vi "Outputs SW Set.vi"(7 "Current Time":timestamp format="%<%x %.3X>T", 8 "Grabber Config":T1={"Grabber Ver"=0, "CAN"={"ID"=0, "Bus"=""}, "Output"={"Type"=enum."Counter-Clockwise", "Neutral"=enum."Override to Coast", "Max"={"FWD"=1.0, "REV"=-1.0}, "Min"={"FWD"=0.0, "REV"=0.0}, "OL Ramp Rate (S)"=0.0, "Dead Band"=0.0}, "StatorLimit"={"Enable"=FALSE, "Current Limit"=0.0, "Threshold Current"=0.0, "Threshold Time"=0.0}} {"Output"."Min"."REV" format="%.2f"; "Output"."Min"."FWD" format="%.2f"; "Output"."Max"."REV" format="%.2f"; "Output"."Max"."FWD" format="%.2f"}, 9 "SW Config":T8={"GrabberSW Ver"=0, "Intake Speed"=0.2, "Eject Speed"=0.2, "Current Limit Velocity"=0, "Current Limit"=6.0, "Current Starting"=20.0, "Max Full Time(S)"=20.0}, 10 "Sensor Values":T10, 11 "SW Output":T9) -> (3 "SW Output Out":T9)   [LabVIEW 2020, in "Grabber_ACT.lvlib"]
uses:
  Grabber_ACT.lvlib
  Shared Code/TypeDefs/Cluster_Grabber HW Outputs.ctl
  Shared Code/TypeDefs/Cluster_FX Sensor Values.ctl
  Shared Code/TypeDefs/Cluster_FX CloseLoop Values.ctl
  Shared Code/TypeDefs/Cluster_FX Current Values.ctl
  Shared Code/TypeDefs/Cluster_Grabber_SW Outputs.ctl
  Shared Code/TypeDefs/Cluster_Grabber_Config SW Values.ctl
  Shared Code/TypeDefs/Cluster_Grabber_Config FX Values.ctl
  Shared Code/TypeDefs/Cluser_CAN Data.ctl
  Shared Code/TypeDefs/Cluster_Config Motor Output.ctl
  <vilib>/Rock Robotics/WPI/ThirdParty/Phoenix-LabVIEW/Motor Controller/Controls/CTRE_Phoenix_MotorControl_TalonFXInvertType.ctl
  <vilib>/Rock Robotics/WPI/ThirdParty/Phoenix-LabVIEW/Motor Controller/Controls/CTRE_Phoenix_MotorControl_NeutralMode.ctl
  Shared Code/TypeDefs/Cluster_FWD  REV Values.ctl
  Shared Code/TypeDefs/Cluser_Config_Current Limits.ctl
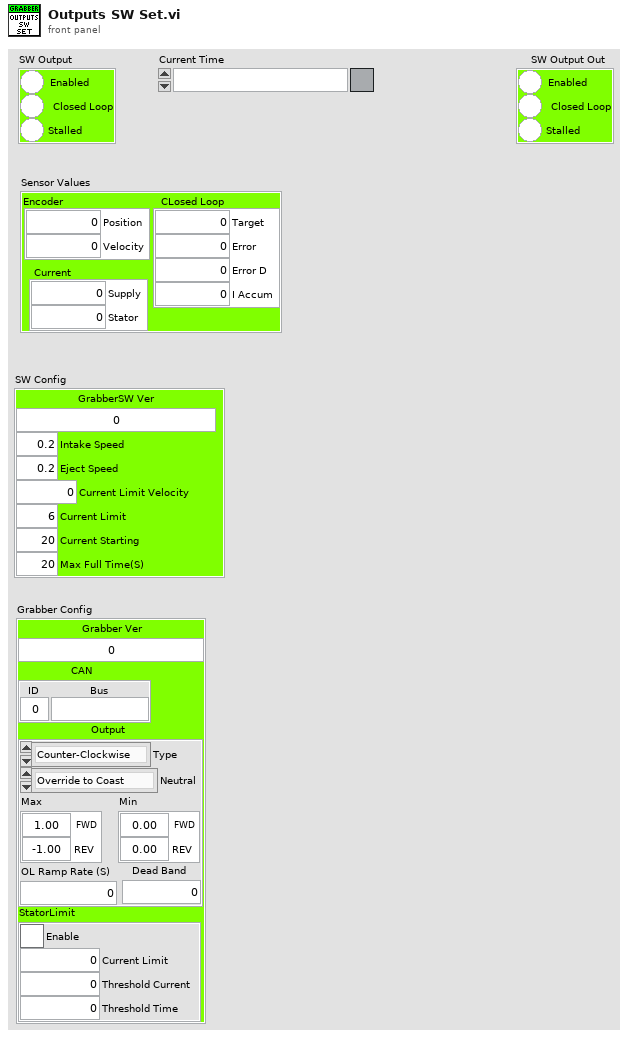
[diagram p1: front panel]
types:
  T1 = typedef "Cluster_Grabber_Config FX Values.ctl" = cluster{"Grabber Ver":u64, "CAN":T2, "Output":T3, "StatorLimit":T7}
  T2 = typedef "Cluser_CAN Data.ctl" = cluster{"ID":u8, "Bus":string}
  T3 = typedef "Cluster_Config Motor Output.ctl" = cluster{"Type":T4, "Neutral":T5, "Max":T6, "Min":T6, "OL Ramp Rate (S)":dbl, "Dead Band":dbl}
  T4 = typedef "CTRE_Phoenix_MotorControl_TalonFXInvertType.ctl" = enum16{"Counter-Clockwise", "Clockwise"}
  T5 = typedef "CTRE_Phoenix_MotorControl_NeutralMode.ctl" = enum8{"EEPROMSetting", "Override to Coast", "Override to Brake"}
  T6 = typedef "Cluster_FWD  REV Values.ctl" = cluster{"FWD":dbl, "REV":dbl}
  T7 = typedef "Cluser_Config_Current Limits.ctl" = cluster{"Enable":bool, "Current Limit":dbl, "Threshold Current":dbl, "Threshold Time":dbl}
  T8 = typedef "Cluster_Grabber_Config SW Values.ctl" = cluster{"GrabberSW Ver":u64, "Intake Speed":dbl, "Eject Speed":dbl, "Current Limit Velocity":i32, "Current Limit":dbl, "Current Starting":dbl, "Max Full Time(S)":dbl}
  T9 = typedef "Cluster_Grabber_SW Outputs.ctl" = cluster{"Enabled":bool, "Closed Loop":bool, "Stalled":bool}
  T10 = typedef "Cluster_Grabber HW Outputs.ctl" = cluster{"Encoder":T11, "CLosed Loop":T12, "Current":T13}
  T11 = typedef "Cluster_FX Sensor Values.ctl" = cluster{"Position":i32, "Velocity":i32}
  T12 = typedef "Cluster_FX CloseLoop Values.ctl" = cluster{"Target":dbl, "Error":i32, "Error D":dbl, "I Accum":dbl}
  T13 = typedef "Cluster_FX Current Values.ctl" = cluster{"Supply":dbl, "Stator":dbl}
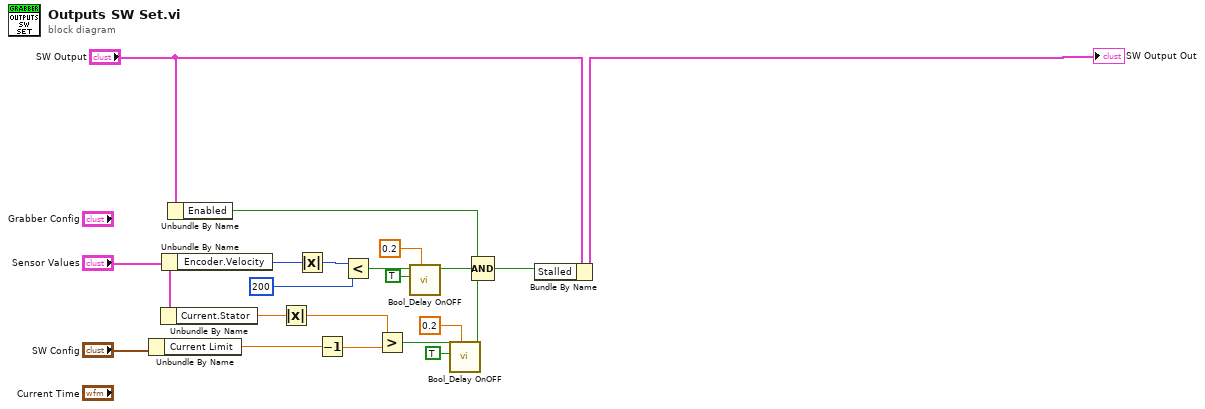
[diagram p0: block diagram]
diagram:
  n1 = Unbundle By Name("SW Config") -> ("Current Limit"=w15:dbl)
  n2 = Unbundle By Name("Sensor Values") -> ("Current.Stator"=w13:dbl)
  n3 = Unbundle By Name("Sensor Values") -> ("Encoder.Velocity"=w21:i32)
  n4 = Unbundle By Name("SW Output") -> ("Enabled"=w3:bool)
  n5 = Absolute Value(x=w13) -> (abs(x)=w1:dbl)
  n6 = Absolute Value(x=w21) -> (abs(x)=w2:i32)
  n7 = Decrement(x=w15) -> (x-1=w12:dbl)
  n8 = Less?(x=w2, y=200) -> (x < y?=w19:bool)
  n9 = Greater?(x=w1, y=w12) -> (0:w9:bool)
  n10 = call "Bool_Delay OnOFF.vi"("Delay Time(S)"=0.2, "Delay On(t) Off(f)"=TRUE, "Input"=w19) -> ("Output"=w8:bool)  [unwired: 7 in, 1 out]
  n11 = call "Bool_Delay OnOFF.vi"("Delay Time(S)"=0.2, "Delay On(t) Off(f)"=TRUE, "Input"=w9) -> ("Output"=w7:bool)  [unwired: 7 in, 1 out]
  n12 = Compound Arithmetic op=AND(w3, w8, w7) -> (w5:bool)
  n13 = Bundle By Name(cluster="SW Output", "Stalled"=w5) -> (→"SW Output Out":T9)
